vi "serialization tests.vi"() -> ()   [LabVIEW 2013, in "dds tests.lvlib"]
uses:
  dds tests.lvlib
  module/configuration/DDS configuration.lvclass
  module/configuration/DDS configuration.lvclass/DDS configuration.ctl
  <vilib>/NI/Tag Bus Module Framework/channel/TBM channel.lvclass
panel:
  out "lines equal 2":bool
  out "lines equal":bool
  out "modules equal":bool
  out "channels equal":bool
  out "no error":errorcluster
  out "no error":errorcluster
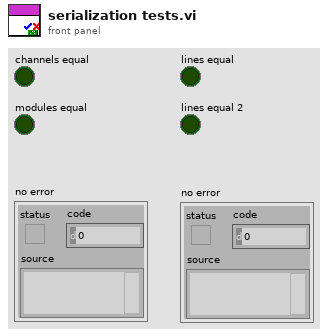
[diagram p1: front panel]
types:
  T1 = typedef "DDS configuration.lvclass/Line.ctl" = cluster{"channel":refnum<class "TBM channel.lvclass">, "DDS topic":string, "DDS Domain":u32, "advanced configuration":T2}
  T2 = typedef "LVDDS_library.lvlib/RTI DDS Advanced Reader Configuration.ctl" = cluster{"typeName":string, "keyName":string, "domainParticipantQoSProfile":string, "dataReaderQoSProfile":string, "forceNewDomainParticipant?":bool, "forceArrayMapping?":bool, "forceExclusiveReader?":bool, "forceRead? (only ExclusiveReader)":bool, "forceUnboundedString?":bool}
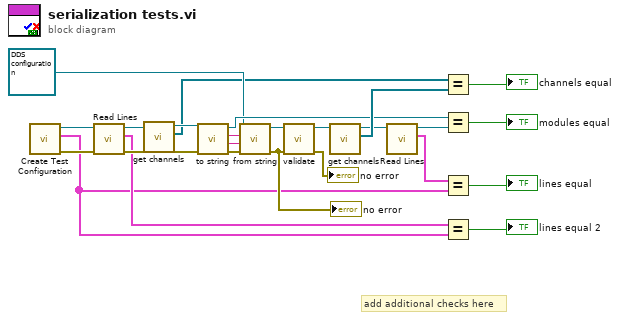
[diagram p0: block diagram]
diagram:
  # "add additional checks here"
  n1 = call "Create Test Configuration.vi"() -> ("error out"=w7:errorcluster, "Line Array"=w1:T1[], "module"=w5:refnum<class "DDS configuration.lvclass">)  [unwired: 6 in, 3 out]
  n2 = call "Read Lines.vi"("error in (no error)"=w7, "dds configuration in"=w5) -> ("error out"=w6:errorcluster, "Lines"=w2:T1[], "dds configuration out"=w4:refnum<class "DDS configuration.lvclass">)  [unwired: 7 in]
  n3 = call-dynamic "get channels.vi"("dds configuration in"=w4) -> ("channels"=w12:refnum<class "TBM channel.lvclass">[], "dds configuration out"=w13:refnum<class "DDS configuration.lvclass">)  [unwired: 9 in]
  n4 = call-dynamic "to string.vi"("error in"=w6, "dds configuration in"=w13) -> ("error out"=w25:errorcluster, "data"=w24:string, "version"=w23:string, "dds configuration out"=w15:refnum<class "DDS configuration.lvclass">)  [unwired: 6 in]
  n5 = call-dynamic "from string.vi"("error in"=w25, "data"=w24, "version"=w23, "dds configuration in"=refnum<class "DDS configuration.lvclass"> refnum ("tag bus configurable plugin module configuration")) -> ("error out"=w20:errorcluster, "dds configuration out"=w22:refnum<class "DDS configuration.lvclass">)  [unwired: 6 in]
  "no error" <- w20
  n6 = call-dynamic "validate.vi"("error in"=w20, "dds configuration in"=w22) -> ("error out"=→"no error":errorcluster, "dds configuration out"=w18:refnum<class "DDS configuration.lvclass">)  [unwired: 8 in]
  n7 = call-dynamic "get channels.vi"("dds configuration in"=w18) -> ("channels"=w17:refnum<class "TBM channel.lvclass">[], "dds configuration out"=w11:refnum<class "DDS configuration.lvclass">)  [unwired: 9 in]
  n8 = call "Read Lines.vi"("dds configuration in"=w11) -> ("Lines"=w9:T1[], "dds configuration out"=w10:refnum<class "DDS configuration.lvclass">)  [unwired: 8 in, 1 out]
  n9 = Equal?(x=w12, y=w17) -> (x = y?=→"channels equal":bool)
  n10 = Equal?(x=w15, y=w10) -> (x = y?=→"modules equal":bool)
  n11 = Equal?(x=w9, y=w1) -> (x = y?=→"lines equal":bool)
  n12 = Equal?(x=w2, y=w1) -> (x = y?=→"lines equal 2":bool)
